vi "Socket_Get TCP Pose.vi"() -> ()   [LabVIEW 2018]
panel:
  out "Routine Complete?":bool
  out "Pcap Iteration":i32
  out "Counter":i32
  in  "PcapCapture":string="tshark -i 6 -p -a filesize:125000 -w Pose"
  in  "Folder Save location":path=path "C:/Users/chetan.malpure/CapturePcap Data"
  out "Iteration":i32
  in  "Stop Button":bool
  out "remote address":string="192.168.0.10"
  out "data out":string
  in  "Client Closed":string="The client VI closed the connection."
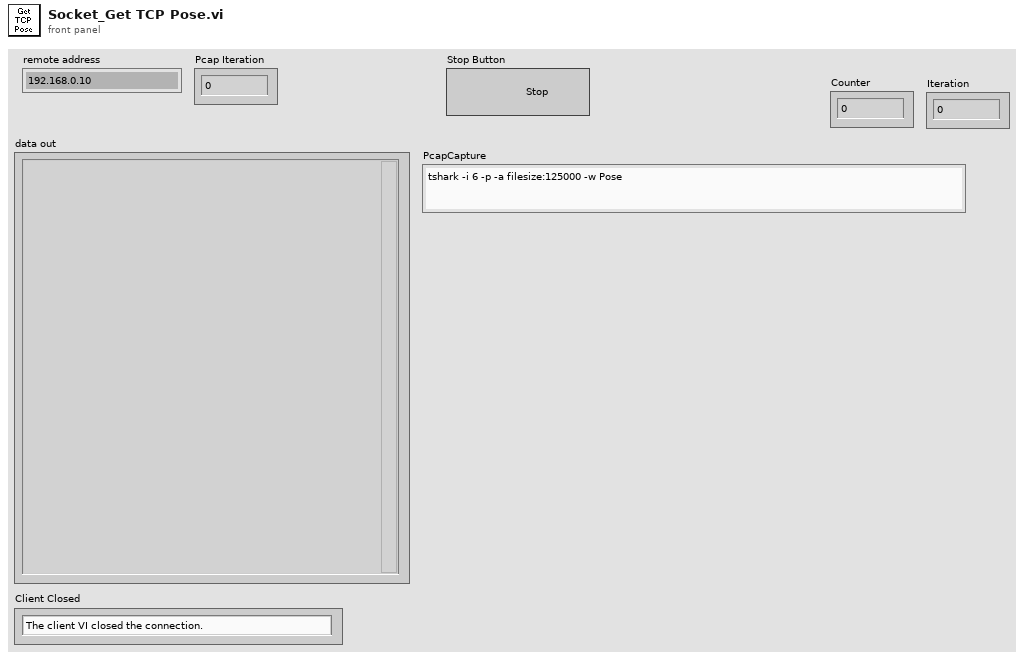
[diagram p1: front panel]
types:
  T1 = enum16{"open", "replace", "create", "open or create", "replace or create", "replace or create with confirmation"}
  T2 = enum16{"Standard", "Buffered", "CRLF", "Immediate"}
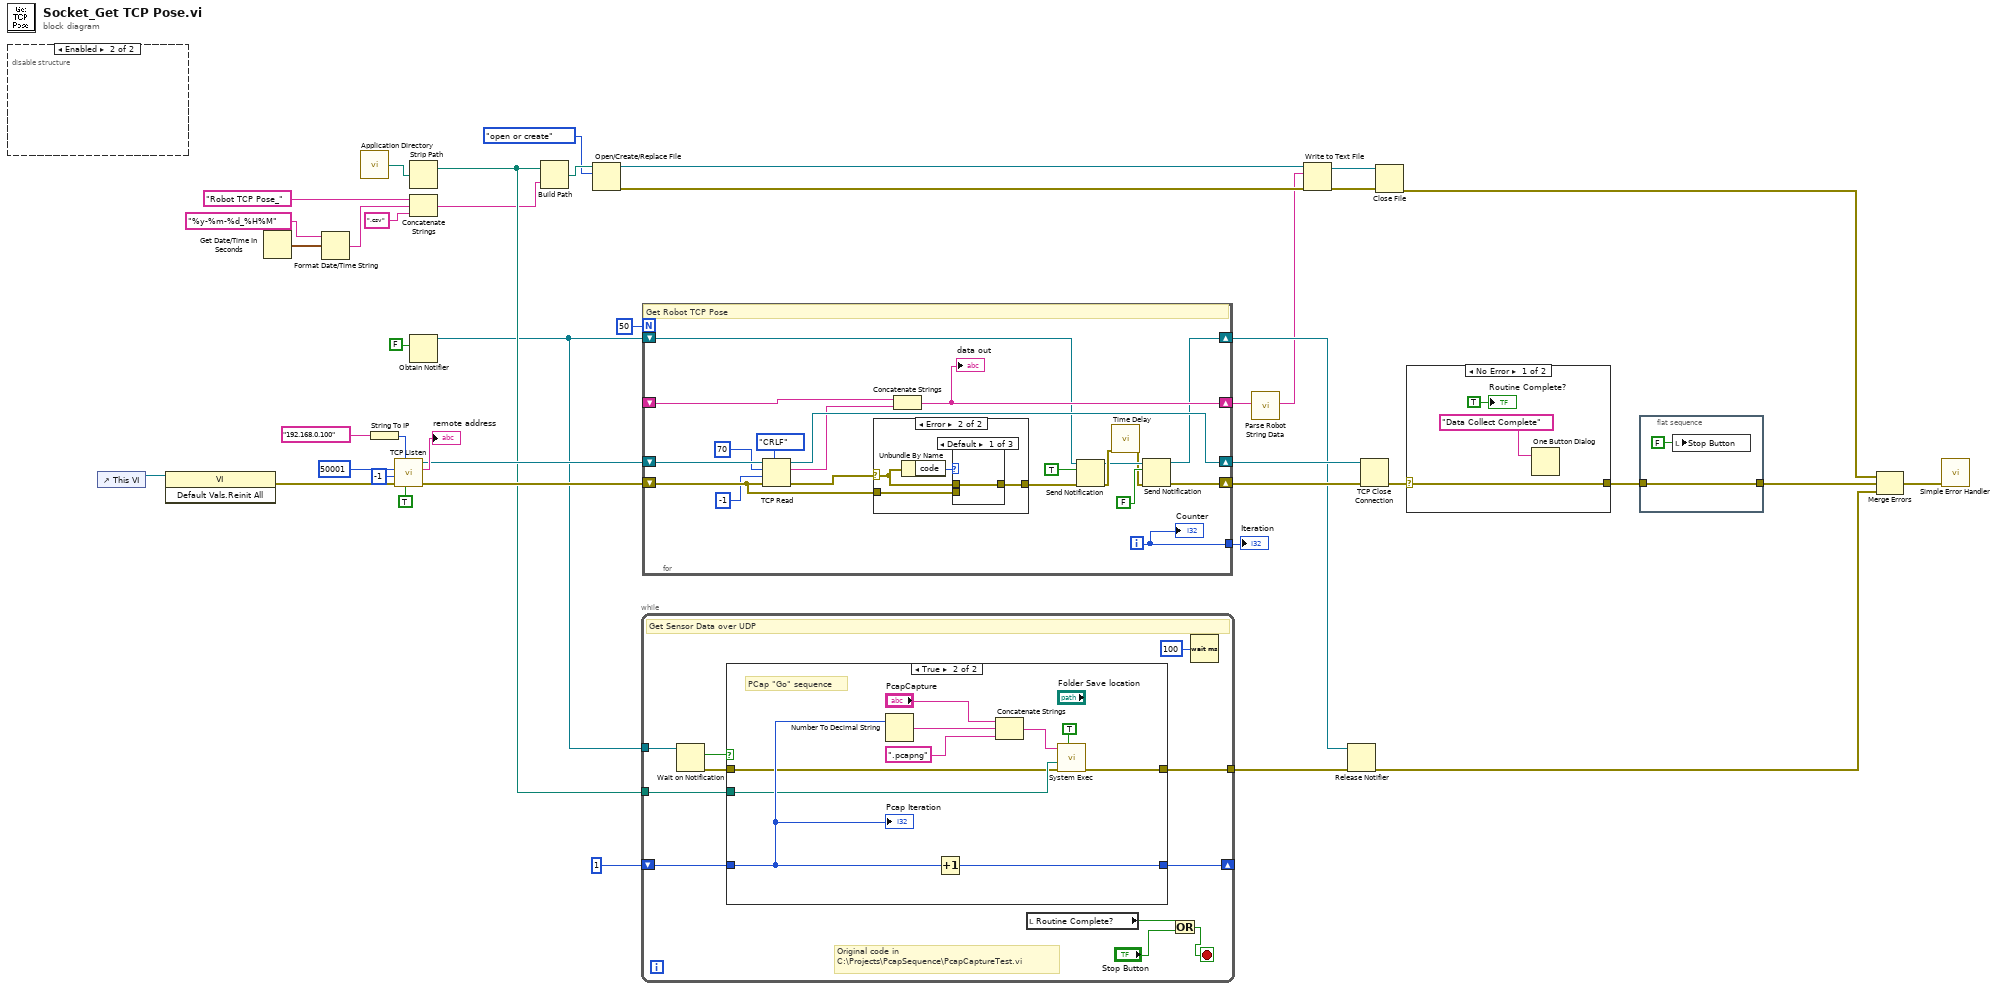
[diagram p0: block diagram]
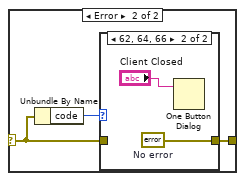
[diagram p6: hidden frame]
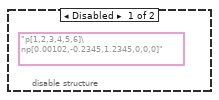
[diagram p8: hidden frame]
diagram:
  n1 = disable-structure shown="Enabled" {
    frame Disabled {
      (unwired) "p[1,2,3,4,5,6]\np[0.00102,-0.2345,1.2345,0,0,0]" ("text")
    }
    frame Enabled {
    }
  }
  n2 = control-ref of="This VI"() -> (w21:refnum<vi>)
  n3 = invoke class="VI" method="Default Vals.Reinit All"(reference=w21) -> (error out=w20:errorcluster)  [unwired: 2 in, 2 out]
  n4 = Get Date/Time In Seconds() -> (seconds since 1Jan1904=w36:timestamp)
  n5 = Format Date/Time String(time format string (%c)="%y-%m-%d_%H%M", seconds (now)=w36) -> (date/time string=w6:string)  [unwired: 1 in]
  n6 = call <vilib>:"Application Directory.vi"() -> ("Application Directory"=w41:path)
  n7 = String To IP(1:"192.168.0.100") -> (0:w27:u32)
  n8 = call <vilib>:"TCP Listen.vi"("resolve remote address (T)"=TRUE, "net address"=w27, "error in (no error)"=w20, "timeout ms (wait forever: -1)"=-1, "port"=u16 50001) -> ("error out"=w29:errorcluster, "remote address"=→"remote address":string, "connection ID"=w24:refnum<k5>)  [unwired: 2 in, 2 out]
  n9 = Strip Path(path=w41) -> (stripped path=w15:path)  [unwired: 1 out]
  n10 = Concatenate Strings("Robot TCP Pose_" ("string"), w6, ".csv" ("string")) -> (w7:string)
  n11 = Obtain Notifier(notification data type=FALSE) -> (notifier out=w13:refnum<notifier>)  [unwired: 3 in, 2 out]
  n12 = Build Path(base path=w15, name or relative path=w7) -> (appended path=w38:path)
  n13 = Open/Create/Replace File(file path (use dialog)=w38, operation (0:open)=T1."open or create") -> (refnum out=w34:refnum<file>, error out=w35:errorcluster)  [unwired: 4 in, 1 out]
  n14 = while {
    shift-right: [w51] -> _
    shift-left: 1 -> [w52]
    tunnel: w15 -> [w50]
    tunnel: w13 -> [w49]
    tunnel: [w47] -> w10
    stop <- w44 stop-if-true
    # "Original code in \nC:\\Projects\\PcapSequence\\PcapCaptureTest.vi"
    # "Get Sensor Data over UDP"
    n15 = Wait on Notification(notifier=w49) -> (notification=w48:bool, error out=w46:errorcluster)  [unwired: 3 in, 2 out]
    n16 = case shown="True" w48 {
      tunnel: w52 -> [w54 w64]
      tunnel: [w54 w63] -> w51
      tunnel: w50 -> [_ w62]
      tunnel: [w53 w56] -> w47
      tunnel: w46 -> [w53 w55]
      frame False {
      }
      frame True {
        # "PCap \"Go\" sequence"
        n17 = Number To Decimal String(number=w64) -> (decimal integer string=w60:string)  [unwired: 1 in]
        n18 = Increment(x=w64) -> (x+1=w63:i32)
        n19 = Concatenate Strings("PcapCapture", w60, ".pcapng" ("string")) -> (w59:string)
        n20 = call <vilib>:"System Exec.vi"("wait until completion? (T)"=TRUE, "error in (no error)"=w55, "working directory"=w62, "command line"=w59) -> ("error out"=w56:errorcluster)  [unwired: 4 in, 3 out]
        "Pcap Iteration" <- w64
      }
    }
    n21 = local read "Routine Complete?"() -> (w42:bool)
    n22 = Or(x=w42, y="Stop Button") -> (x .or. y?=w44:bool)
    n23 = Wait (ms)(milliseconds to wait=u32 100) -> ()  [unwired: 1 out]
  }
  n24 = for {
    N: 50 -> [_]
    shift-right: [w70] -> w22
    shift-left: w29 -> [w84]
    shift-right: [w82] -> w23
    shift-left: w24 -> [w83]
    shift-right: [w77] -> w5
    shift-left: _ -> [w78]
    tunnel: [w76] -> w2
    shift-right: [w68] -> w12
    shift-left: w13 -> [w67]
    i -> [w76]
    # "Get Robot TCP Pose"
    n25 = TCP Read(connection ID=w83, bytes to read=70, error in (no error)=w84, 7:T2."CRLF" ("mode (standard)"), 9:-1 ("timeout ms (25000)")) -> (connection ID out=w82:refnum<k5>, data out=w75:string, error out=w74:errorcluster)
    n26 = case shown="Error" w74 {
      selector: w74 -> [w85 w88]
      tunnel: [w85 w86] -> w73
      tunnel: w84 -> [_ w87]
      frame No Error {
      }
      frame Error {
        n27 = Unbundle By Name(w88) -> ("code"=w89:i32)
        n28 = case shown="Default" w89 {
          tunnel: w88 -> [w90 _ _]
          tunnel: w87 -> [_ w91 w92]
          tunnel: [w90 w91 w92] -> w86
          frame Default {
          }
          frame 56 {
          }
          frame 66 {
          }
        }
      }
    }
    n29 = Concatenate Strings(w78, w75) -> (w77:string)
    "data out" <- w77
    n30 = Send Notification(notification=TRUE, notifier=w67, error in (no error)=w73) -> (notifier out=w66:refnum<notifier>, error out=w71:errorcluster)
    n31 = call "Time Delay"("error in (no error)"=w71) -> ("error out"=w65:errorcluster)  [unwired: 10 in]
    n32 = Send Notification(notification=FALSE, notifier=w66, error in (no error)=w65) -> (notifier out=w68:refnum<notifier>, error out=w70:errorcluster)
    "Counter" <- w76
  }
  "Iteration" <- w2
  n33 = call "Parse Robot String Data.vi"("Str_Robot_TCP_Poses"=w5) -> ("Parsed String Out"=w4:string)  [unwired: 10 in]
  n34 = Write to Text File(file (use dialog)=w34, text=w4, error in=w35) -> (refnum out=w32:refnum<file>, error out=w33:errorcluster)  [unwired: 1 in, 1 out]
  n35 = Release Notifier(notifier=w12, error in (no error)=w10) -> (error out=w9:errorcluster)  [unwired: 1 in, 2 out]
  n36 = TCP Close Connection(connection ID=w23, error in (no error)=w22) -> (error out=w17:errorcluster)  [unwired: 2 out]
  n37 = Close File(refnum=w32, error in=w33) -> (error out=w19:errorcluster)  [unwired: 1 out]
  n38 = case shown="No Error" w17 {
    selector: w17 -> [w95 w97]
    tunnel: [w95 w96] -> w8
    frame No Error {
      n39 = One Button Dialog(message="Data Collect Complete") -> ()  [unwired: 1 in, 1 out]
      "Routine Complete?" <- TRUE ("Routine Complete?")
    }
    frame Error {
      n40 = Unbundle By Name(w97) -> ("code"=w98:i32)
      n41 = case shown="62, 64, 66" w98 {
        tunnel: w97 -> [w99 _]
        tunnel: [w99 w101] -> w96
        frame Default {
        }
        frame 62, 64, 66 {
          w101 = errorcluster {"status"=FALSE, "code"=0, "source"=""}  # No error
          n42 = One Button Dialog(message="Client Closed") -> ()  [unwired: 1 in, 1 out]
        }
      }
    }
  }
  n43 = flat-sequence {
    tunnel: w8 -> [w102]
    tunnel: [w102] -> w11
    frame #0 {
      n44 = local write "Stop Button"(FALSE ("Stop Button")) -> ()
    }
  }
  n45 = Merge Errors(w19, w11, w9) -> (w18:errorcluster)
  n46 = call <vilib>:"Simple Error Handler.vi"("error in (no error)"=w18) -> ()  [unwired: 1 in, 8 out]
